vi "Evaluate Bytewise 16bit checksum.vi"(7 "End Offset  for Checksum Calc":i32=-2, 8 "Start Offset for Checksum Calc":i32, 9 "Intput String":string) -> (0 "Output String with Checksum":string, 1 "Checksum as Calculated":u16 format="%.0x", 2 "Checksum Error":bool, 3 "Output String":string)   [LabVIEW 2017]
panel:
  out "Checksum as Read":u16 format="%.0x"
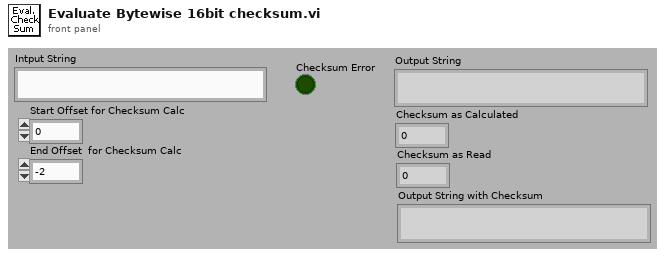
[diagram p1: front panel]
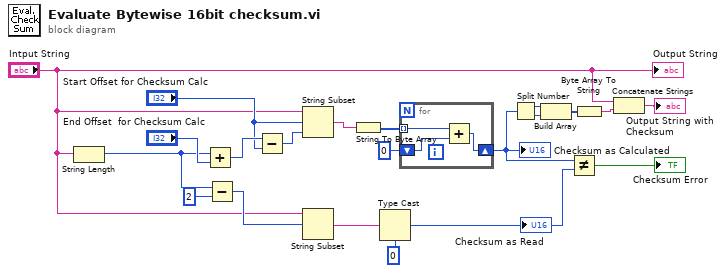
[diagram p0: block diagram]
diagram:
  n1 = String Length(string="Intput String") -> (length=w12:i32)
  n2 = Add(x=w12, y="End Offset  for Checksum Calc") -> (x+y=w10:i32)
  n3 = Subtract(x=w12, y=2) -> (x-y=w13:i32)
  n4 = Subtract(x=w10, y="Start Offset for Checksum Calc") -> (x-y=w8:i32)
  n5 = String Subset(string="Intput String", offset (0)="Start Offset for Checksum Calc", length (rest)=w8) -> (substring=w16:string)
  n6 = String Subset(string="Intput String", offset (0)=w13) -> (substring=w15:string)  [unwired: 1 in]
  n7 = String To Byte Array(string=w16) -> (unsigned byte array=w19:u8[])
  n8 = Type Cast(type=u16 0, x=w15) -> (*(type *) &x=w21:u16)
  "Checksum as Read" <- w21
  n9 = for {
    shift-right: [w24] -> w1
    shift-left: u16 0 -> [w22]
    tunnel: w19 -> [w23] mode=indexing
    n10 = Add(x=w23, y=w22) -> (x+y=w24:u16)
  }
  "Checksum as Calculated" <- w1
  n11 = Split Number(x=w1) -> (hi(x)=w5:u8, lo(x)=w4:u8)
  n12 = Build Array(w5, w4) -> (w3:u8[])
  n13 = Not Equal?(x=w1, y=w21) -> (x != y?=→"Checksum Error":bool)
  n14 = Byte Array To String(unsigned byte array=w3) -> (string=w2:string)
  n15 = Concatenate Strings("Intput String", w2) -> (→"Output String with Checksum":string)
  "Output String" <- "Intput String"
